vi "SimpleRegAndResolve.vi"() -> ()   [LabVIEW 2024, in "Module Container.lvlib"]
uses:
  Module Container.lvlib
  Module/RQMHModule.lvclass
  Scripting/templates/TemplateModule/TemplateModule.lvclass
  JQMHStartup/RQMHStartup.lvclass
panel:
  out "Already Running":bool
  out "error out":errorcluster
  in  "stop":bool
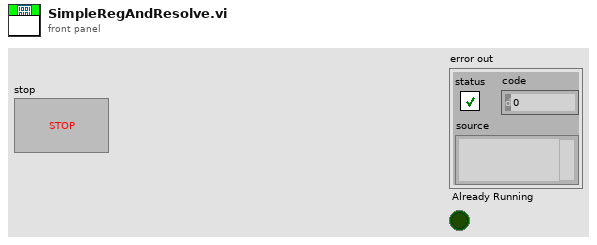
[diagram p1: front panel]
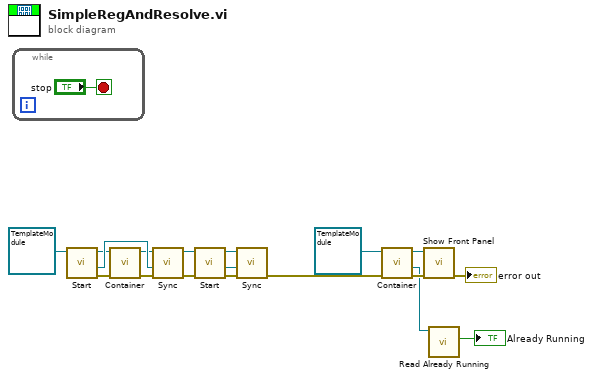
[diagram p0: block diagram]
diagram:
  n1 = while {
    stop <- "stop" stop-if-true
  }
  n2 = call "Start.vi"("JQMHCore in"=refnum<class "TemplateModule.lvclass"> refnum ("TemplateModule.lvclass")) -> ("error out"=w7:errorcluster, "StartupHandshake out"=w18:refnum<class "RQMHStartup.lvclass">, "JQMHCore out"=w12:refnum<class "TemplateModule.lvclass">)  [unwired: 8 in]
  n3 = call "Container.vi"("error in (no error)"=w7, "Module Type"=w12) -> ("error out"=w6:errorcluster, "Module Instance"=w11:refnum<class "TemplateModule.lvclass">)  [unwired: 7 in, 1 out]
  n4 = call "Sync.vi"("error in (no error)"=w6, "StartupHandshake out"=w18, "JQMHCore in"=w11) -> ("error out"=w5:errorcluster, "JQMHCore out"=w15:refnum<class "TemplateModule.lvclass">)  [unwired: 7 in]
  n5 = call "Start.vi"("error in (no error)"=w5, "JQMHCore in"=w15) -> ("error out"=w16:errorcluster, "StartupHandshake out"=w13:refnum<class "RQMHStartup.lvclass">, "JQMHCore out"=w14:refnum<class "TemplateModule.lvclass">)  [unwired: 7 in]
  n6 = call "Sync.vi"("error in (no error)"=w16, "StartupHandshake out"=w13, "JQMHCore in"=w14) -> ("error out"=w9:errorcluster)  [unwired: 7 in, 1 out]
  n7 = call "Container.vi"("error in (no error)"=w9, "Module Type"=refnum<class "TemplateModule.lvclass"> refnum ("TemplateModule.lvclass")) -> ("error out"=w4:errorcluster, "Handshake (if started)"=w2:refnum<class "RQMHStartup.lvclass">, "Module Instance"=w8:refnum<class "TemplateModule.lvclass">)  [unwired: 7 in]
  n8 = call "Show Front Panel.vi"("error in (no error)"=w4, "JQMHCore in"=w8) -> ("error out"=→"error out":errorcluster)  [unwired: 8 in, 1 out]
  n9 = call "Read Already Running.vi"("JQMHStartup in"=w2) -> ("Already Running"=→"Already Running":bool)  [unwired: 9 in, 1 out]
